vi "Dibuix_pistola.vi"(8 "Esquerra/Dreta (-1/1)":dbl, 11 "Posició Y":dbl) -> (3 "Dibuix pistola":cluster{dbl[], dbl[]}={[-0.99, -0.985, -0.98, -0.975, -0.86, -0.88, -0.9, -0.92, -0.94, -0.96, -0.98, -1.0, -0.94, -0.96, -0.98, -0.86], [-4.0, -3.0, -2.0, -1.0, 0.0, 0.0, 0.0, 0.0, 0.0, 0.0, 0.0, 0.0, -1.0, -2.0, -3.0, 0.5]})   [LabVIEW 2020]
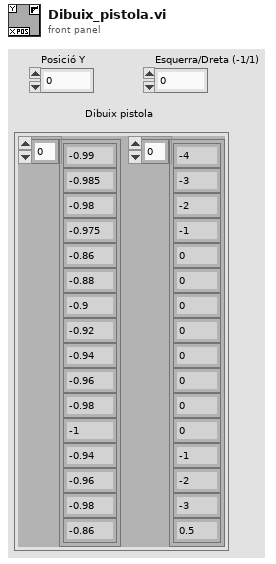
[diagram p1: front panel]
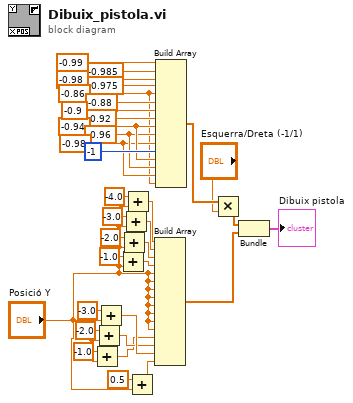
[diagram p0: block diagram]
diagram:
  w6 = -0.86
  w11 = -0.94
  w10 = -0.96
  w9 = -0.98
  n1 = Add(x=-1.0, y="Posició Y") -> (x+y=w12:dbl)
  n2 = Add(x=-2.0, y="Posició Y") -> (x+y=w13:dbl)
  n3 = Add(x=-3.0, y="Posició Y") -> (x+y=w14:dbl)
  n4 = Add(x=-1.0, y="Posició Y") -> (x+y=w26:dbl)
  n5 = Add(x=-2.0, y="Posició Y") -> (x+y=w25:dbl)
  n6 = Add(x=-3.0, y="Posició Y") -> (x+y=w24:dbl)
  n7 = Add(x=-4.0, y="Posició Y") -> (x+y=w30:dbl)
  n8 = Add(x=0.5, y="Posició Y") -> (x+y=w7:dbl)
  n9 = Build Array(w30, w24, w25, w26, "Posició Y", "Posició Y", "Posició Y", "Posició Y", "Posició Y", "Posició Y", "Posició Y", "Posició Y", w12, w13, w14, w7) -> (w34:dbl[])
  n10 = Build Array(-0.99, -0.985, -0.98, -0.975, w6, -0.88, -0.9, -0.92, w11, w10, w9, -1, w11, w10, w9, w6) -> (w3:dbl[])
  n11 = Multiply(x=w3, y="Esquerra/Dreta (-1/1)") -> (x*y=w2:dbl[])
  n12 = Bundle(w2, w34) -> (→"Dibuix pistola":cluster{dbl[], dbl[]})  [unwired: 1 in]
